vi "Read.vi"(8 "error in (no error)":errorcluster, 9 "Variant":variant, 11 "VISA in":refnum<class "VISA.lvclass">) -> (0 "error out":errorcluster, 2 "String":string, 3 "VISA out":refnum<class "VISA.lvclass">)   [LabVIEW 2019, in "Protocols.lvlib" / "VISA.lvclass"]
uses:
  VISA.lvclass
  Protocol Parent/Methods/Read Parameter.ctl
  VISA.lvclass/VISA.ctl
  Read Ref.vi
  Write Ref.vi
  <vilib>/Utility/error.llb/Clear Errors.vi
  Protocol Parent/Protocol Parent.lvclass
  Protocols.lvlib
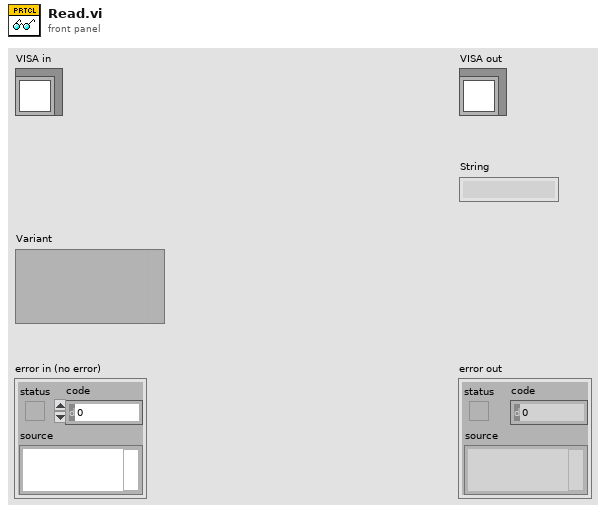
[diagram p1: front panel]
types:
  T1 = typedef "Protocols.lvlib/Protocol Parent.lvclass/Read Parameter.ctl" = cluster{"Wait Type":enum16{"Byte Count", "Wait sec"}, "Wait Value":dbl}
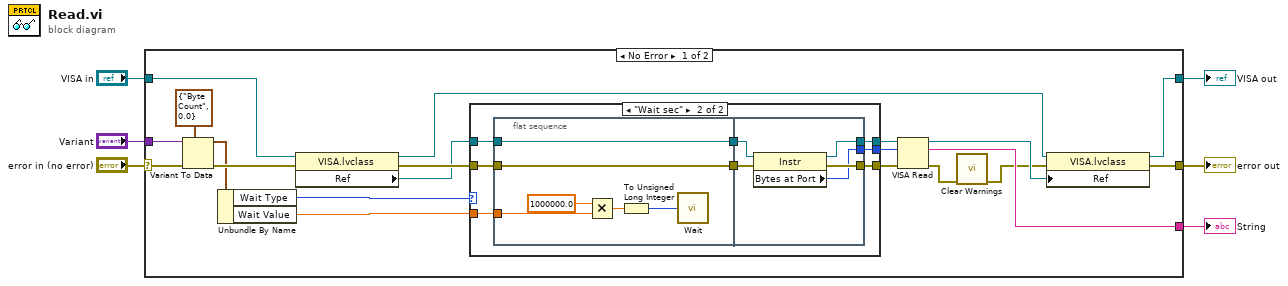
[diagram p0: block diagram]
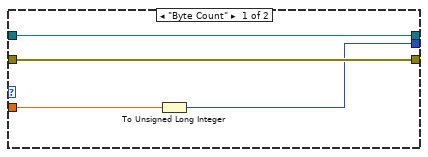
[diagram p2: hidden frame]
diagram:
  n1 = case shown="No Error" "error in (no error)" {
    selector: "error in (no error)" -> [w21 w51]
    tunnel: "VISA in" -> [w26 w50]
    tunnel: [w24 w51] -> w3
    tunnel: [w22 w50] -> w1
    tunnel: "Variant" -> [w19 _]
    tunnel: [w10 _] -> w2
    frame No Error {
      n2 = Variant To Data(error in=w21, type=T1 {"Wait Type"=enum."Byte Count", "Wait Value"=0.0} ("Read Parameter"), Variant=w19) -> (data=w18:T1, error out=w20:errorcluster)
      n3 = Unbundle By Name(w18) -> ("Wait Type"=w12:enum16{"Byte Count", "Wait sec"}, "Wait Value"=w11:dbl)
      n4 = property class="VISA.lvclass"(reference=w26, error in=w20) -> (reference out=w23:refnum<class "VISA.lvclass">, error out=w17:errorcluster, "Ref"=w16:refnum<visa-resource-name>)
      n5 = case shown="\"Wait sec\"" w12 {
        tunnel: w17 -> [w30 w38]
        tunnel: w16 -> [w29 w37]
        tunnel: [w30 w36] -> w15
        tunnel: [w29 w35] -> w14
        tunnel: [w27 w34] -> w13
        tunnel: w11 -> [w28 w31]
        frame "Byte Count" {
          n6 = To Unsigned Long Integer(number=w28) -> (unsigned 32bit integer=w27:u32)
        }
        frame "Wait sec" {
          n7 = flat-sequence {
            tunnel: w37 -> [w43]
            tunnel: w38 -> [w44]
            tunnel: [w44] -> w33
            tunnel: [w43] -> w32
            tunnel: w31 -> [w40]
            tunnel: [w47] -> w36
            tunnel: [w46] -> w35
            tunnel: [w45] -> w34
            tunnel: w33 -> [w49]
            tunnel: w32 -> [w48]
            frame #0 {
              n8 = Multiply(x=1000000.0, y=w40) -> (x*y=w42:dbl)
              n9 = To Unsigned Long Integer(number=w42) -> (unsigned 32bit integer=w39:u32)
              n10 = call "Wait"("Count(uSec)"=w39) -> ()  [unwired: 1 out]
            }
            frame #1 {
              n11 = property class="Instr"(reference=w48, error in=w49) -> (reference out=w46:refnum<visa-resource-name>, error out=w47:errorcluster, "Bytes at Port"=w45:u32)
            }
          }
        }
      }
      n12 = VISA Read(VISA resource name=w14, byte count=w13, error in (no error)=w15) -> (VISA resource name out=w25:refnum<visa-resource-name>, read buffer=w10:string, error out=w8:errorcluster)  [unwired: 1 out]
      n13 = call "Clear Warnings.vi"("error in (no error)"=w8) -> ("error out"=w7:errorcluster)  [unwired: 10 in]
      n14 = property class="VISA.lvclass"(reference=w23, error in=w7, "Ref"=w25) -> (reference out=w22:refnum<class "VISA.lvclass">, error out=w24:errorcluster)
    }
    frame Error {
    }
  }
  "error out" <- w3
  "VISA out" <- w1
  "String" <- w2
